vi "HXG2_TableFormattingForActiveTestPoint.vi"(7 "Current Step":i32=-1, 8 "error IO":errorcluster, 11 "Table Control":refnum<vi>) -> (0 "error out":errorcluster, 3 "Current Step Out":i32)   [LabVIEW 2012]
doc: "Format table to highlight current test point"
uses:
  <vilib>/Utility/miscctls.llb/LVRowAndColumnTypeDef.ctl
  <vilib>/Utility/miscctls.llb/LVBoundsTypeDef.ctl
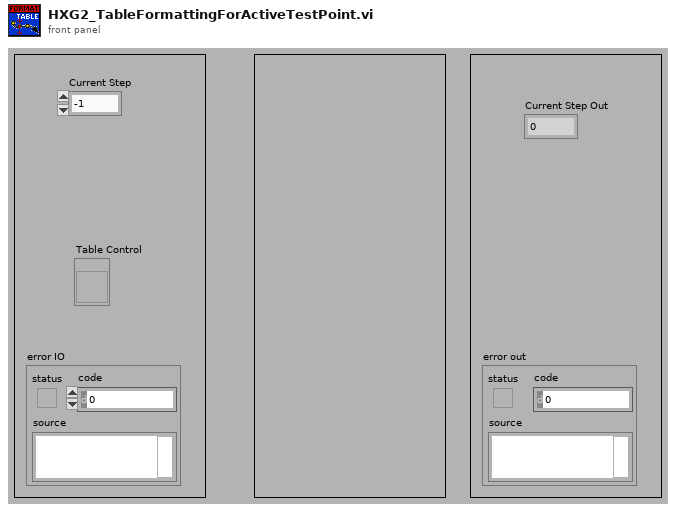
[diagram p1: front panel]
types:
  T1 = typedef "LVBoundsTypeDef.ctl" = cluster{"Width":u32, "Height":u32}
  T2 = typedef "LVRowAndColumnTypeDef.ctl" = cluster{"Row":i32, "Column":i32}
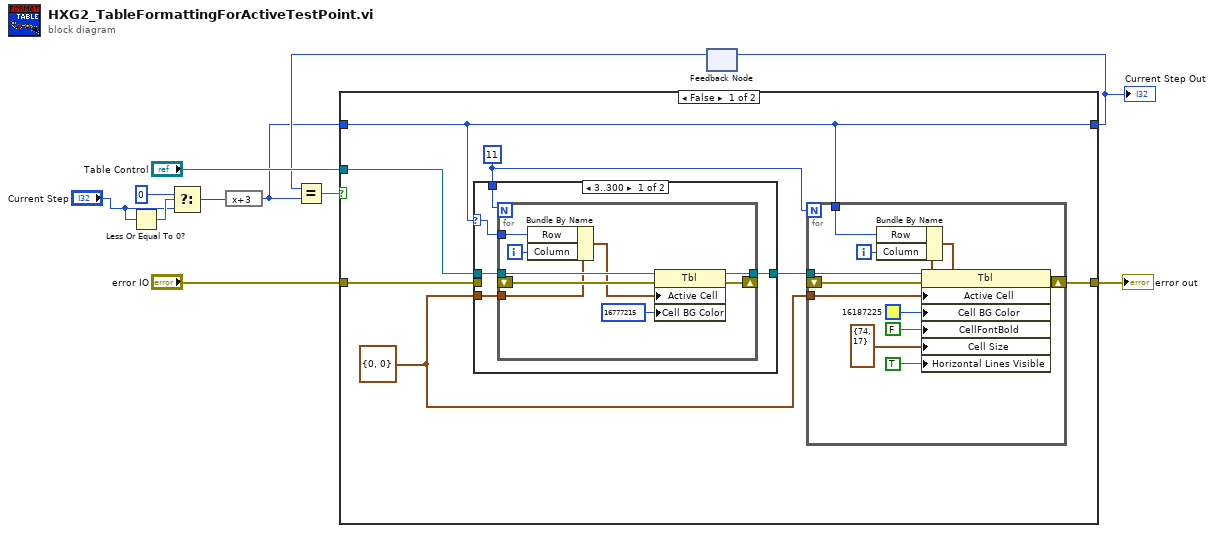
[diagram p0: block diagram]
diagram:
  n1 = Less Or Equal To 0?(x="Current Step") -> (x <= 0?=w4:bool)
  n2 = Select(t=0, s=w4, f="Current Step") -> (s? t:f=w1:i32)
  n3 = expression code="x+3"(w1) -> (w5:i32)
  n4 = feedback #1() -> (w6:i32)  [unwired: 1 in]
  n5 = Equal?(x=w6, y=w5) -> (x = y?=w10:bool)
  n6 = case shown="False" w10 {
    tunnel: [w18 w45] -> w7
    tunnel: w5 -> [w12 w46]
    tunnel: [w12 w46] -> w11
    tunnel: "error IO" -> [w16 w45]
    tunnel: "Table Control" -> [w17 _]
    frame False {
      w15 = 11
      w13 = T2 {"Row"=0, "Column"=0} ("Active Cell:Active Cell")
      n7 = case shown="3..300" w12 {
        selector: w12 -> [w19 _]
        tunnel: w17 -> [w21 w33]
        tunnel: w16 -> [_ _]
        tunnel: w13 -> [w22 _]
        tunnel: w15 -> [w23 _]
        tunnel: [w20 w33] -> w14
        frame 3..300 {
          n8 = for {
            N: w23 -> [_]
            tunnel: w21 -> [w32]
            tunnel: w22 -> [w29]
            shift-right: [w30] -> _
            shift-left: _ -> [w31]
            tunnel: [w26] -> w20
            tunnel: w19 -> [w25]
            i -> [w28]
            n9 = Bundle By Name(cluster=w29, "Row"=w25, "Column"=w28) -> (w27:T2)
            n10 = property class="Tbl"(reference=w32, error in=w31, "Active Cell"=w27, "Cell BG Color"=u32 16777215 ("y")) -> (reference out=w26:refnum<vi>, error out=w30:errorcluster)
          }
        }
        frame 0..2, Default {
        }
      }
      n11 = for {
        N: w15 -> [_]
        tunnel: w14 -> [w44]
        tunnel: w13 -> [w41]
        shift-right: [w42] -> w18
        shift-left: _ -> [w43]
        tunnel: w12 -> [w37]
        i -> [w40]
        n12 = Bundle By Name(cluster=w41, "Row"=w37, "Column"=w40) -> (w39:T2)
        n13 = property class="Tbl"(reference=w44, error in=w43, "Active Cell"=w39, "Cell BG Color"=u32 16187225, "CellFontBold"=FALSE ("Active Cell:Cell Font:Bold"), "Cell Size"=T1 {"Width"=74, "Height"=17} ("Active Cell:Cell Size"), "Horizontal Lines Visible"=TRUE ("Active Cell:Cell Font:Bold")) -> (error out=w42:errorcluster)  [unwired: 1 out]
      }
    }
    frame True {
    }
  }
  "error out" <- w7
  "Current Step Out" <- w11
  n14 = feedback-in #1(w11) -> ()
